vi "Add Default Free.vi"(8 "error in (no error)":errorcluster, 10 "ToModBus":bool, 11 "Tach In":refnum<class "Tachometer.lvclass">) -> (0 "error out":errorcluster, 3 "Tach Out":refnum<class "Tachometer.lvclass">)   [LabVIEW 2018, in "Measurement Channels.lvlib" / "Tachometer.lvclass"]
uses:
  Tachometer.lvclass
  C:/Users/Jeff Tipps/Documents/DAQMan/source/Classes/Measurements/Class Channel/Channel.lvclass
  C:/Users/Jeff Tipps/Documents/DAQMan/source/Classes/Measurements/Class Frequency/Frequency.lvclass
  Tachometer.lvclass/Tachometer.ctl
  Class Channel/Write Unit_EU.vi
  Class Frequency/Write Min EU.vi
  Class Frequency/Frequency.lvclass
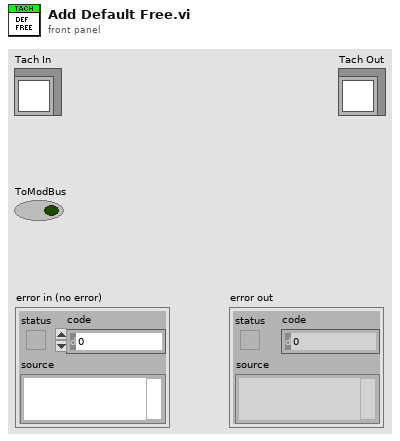
[diagram p1: front panel]
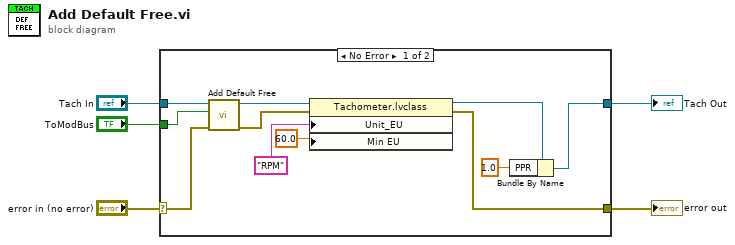
[diagram p0: block diagram]
diagram:
  n1 = case shown="No Error" "error in (no error)" {
    selector: "error in (no error)" -> [w13 w18]
    tunnel: "Tach In" -> [w14 w17]
    tunnel: [w16 w17] -> w5
    tunnel: [w7 w18] -> w4
    tunnel: "ToModBus" -> [w12 _]
    frame No Error {
      n2 = call-parent "Add Default Free.vi"("error in (no error)"=w13, "ToModBus"=w12, "Frequency"=w14) -> ("error out"=w10:errorcluster, "Frequency Out"=w11:refnum<class "Tachometer.lvclass">)  [unwired: 7 in]
      n3 = property class="Tachometer.lvclass"(reference=w11, error in=w10, "Unit_EU"="RPM", "Min EU"=60.0) -> (reference out=w8:refnum<class "Tachometer.lvclass">, error out=w7:errorcluster)
      n4 = Bundle By Name(cluster=w8, "PPR"=1.0) -> (w16:refnum<class "Tachometer.lvclass">)
    }
    frame Error {
    }
  }
  "Tach Out" <- w5
  "error out" <- w4
